vi "Validate Payload Times.vi"(11 "Payload":string) -> (3 "Times Valid":bool)   [LabVIEW 2020, in "JWT.lvlib" / "JWT.lvclass"]
uses:
  JWT.lvclass
  JWT.lvlib
  lv-json/JSON/JSON.lvlib
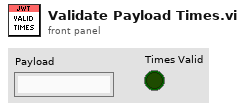
[diagram p1: front panel]
types:
  T1 = typedef "JSON.lvlib/JSON Item Type.ctl" = enum16{"unknown", "null", "Array", "Object", "String", "Number", "Boolean"}
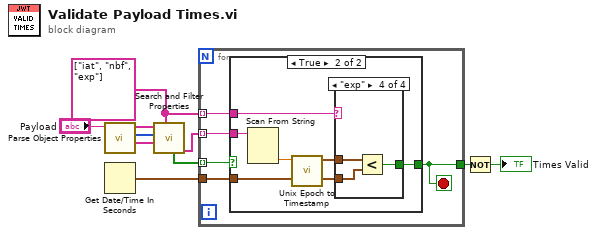
[diagram p0: block diagram]
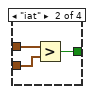
[diagram p4: hidden frame]
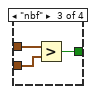
[diagram p5: hidden frame]
diagram:
  w4 = string[] ["iat", "nbf", "exp"] ("Search Keys")
  n1 = call "Parse Object Properties.vi"("JSON String"="Payload") -> ("Values"=w7:string[], "Item Types"=w8:T1[], "Keys"=w9:string[])  [unwired: 7 in, 1 out]
  n2 = Get Date/Time In Seconds() -> (seconds since 1Jan1904=w3:timestamp)
  n3 = call "Search and Filter Properties.vi"("Search Keys"=w4, "Values In"=w7, "Types In"=w8, "Keys In"=w9) -> ("Filtered Values"=w5:string[], "Item Found"=w6:bool[])  [unwired: 2 in, 4 out]
  n4 = for {
    tunnel: w6 -> [w15] mode=indexing
    tunnel: w5 -> [w14] mode=indexing
    tunnel: w4 -> [w13] mode=indexing
    tunnel: w3 -> [w12]
    tunnel: [w11] -> w2
    stop <- w11 stop-if-true
    n5 = case shown="True" w15 {
      tunnel: w14 -> [_ w19]
      tunnel: w13 -> [_ w21]
      tunnel: w12 -> [_ w20]
      tunnel: [_ w16] -> w11
      frame False {
      }
      frame True {
        n6 = Scan From String(input string=w19) -> (output 1=w18:dbl)  [unwired: 4 in, 3 out]
        n7 = call "Unix Epoch to Timestamp.vi"("Unix Epoch Seconds"=w18) -> ("Time Stamp"=w17:timestamp)  [unwired: 9 in, 1 out]
        n8 = case shown="\"exp\"" w21 {
          tunnel: w20 -> [_ w23 w26 w29]
          tunnel: w17 -> [_ w24 w27 w30]
          tunnel: [_ w22 w25 w28] -> w16
          frame Default {
          }
          frame "iat" {
            n9 = Greater?(x=w24, y=w23) -> (0:w22:bool)
          }
          frame "nbf" {
            n10 = Greater?(x=w27, y=w26) -> (0:w25:bool)
          }
          frame "exp" {
            n11 = Less?(x=w30, y=w29) -> (x < y?=w28:bool)
          }
        }
      }
    }
  }
  n12 = Not(x=w2) -> (.not. x?=→"Times Valid":bool)
